vi "Ch_data_pattern_8_save (SubVI).vi"(7 "error in":errorcluster, 14 "T Cluster":T2 {"T8" format="%#.3f"; "T7" format="%#.3f"; "T6" format="%#.3f"; "T5" format="%#.3f"; "T4" format="%#.3f"; "T3" format="%#.3f"; "T2" format="%#.3f"; "T1" format="%#.3f"}, 17 "file":refnum<file>, 18 "R cluster":T1 {"R8" format="%#.3f"; "R7" format="%#.3f"; "R6" format="%#.3f"; "R5" format="%#.3f"; "R4" format="%#.3f"; "R3" format="%#.3f"; "R2" format="%#.3f"; "R1" format="%#.3f"}) -> (27 "error out":errorcluster)   [LabVIEW 2015]
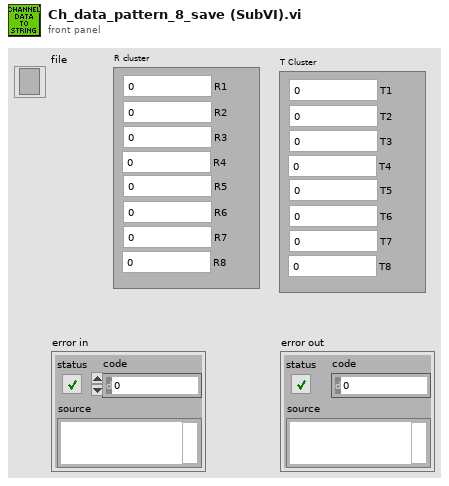
[diagram p1: front panel]
types:
  T1 = cluster{"R1":dbl, "R2":dbl, "R3":dbl, "R4":dbl, "R5":dbl, "R6":dbl, "R7":dbl, "R8":dbl}
  T2 = cluster{"T1":dbl, "T2":dbl, "T3":dbl, "T4":dbl, "T5":dbl, "T6":dbl, "T7":dbl, "T8":dbl}
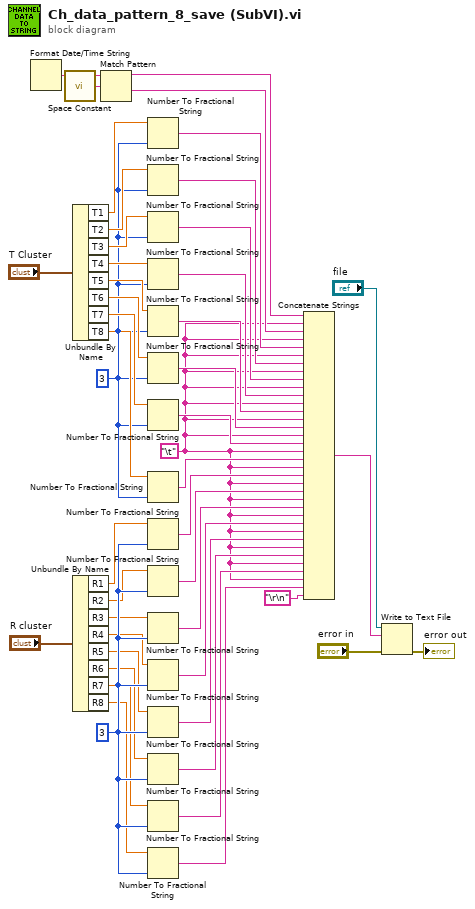
[diagram p0: block diagram]
diagram:
  w19 = i16 3 ("precision (6)")
  w25 = i16 3 ("precision (6)")
  w3 = "\t"
  n1 = Format Date/Time String() -> (date/time string=w44:string)  [unwired: 3 out]
  n2 = call <vilib>:"Space Constant.vi"() -> ("String"=w45:string)
  n3 = Unbundle By Name("T Cluster") -> ("T1"=w33:dbl, "T2"=w32:dbl, "T3"=w31:dbl, "T4"=w30:dbl, "T5"=w29:dbl, "T6"=w28:dbl, "T7"=w27:dbl, "T8"=w26:dbl)
  n4 = Unbundle By Name("R cluster") -> ("R1"=w18:dbl, "R2"=w17:dbl, "R3"=w16:dbl, "R4"=w15:dbl, "R5"=w14:dbl, "R6"=w13:dbl, "R7"=w12:dbl, "R8"=w11:dbl)
  n5 = Match Pattern(string=w44, regular expression=w45) -> (before substring=w37:string, after substring=w36:string)  [unwired: 3 out]
  n6 = Number To Fractional String(number=w33, precision (6)=w25) -> (F-format string=w42:string)  [unwired: 2 out]
  n7 = Number To Fractional String(number=w32, precision (6)=w25) -> (F-format string=w38:string)  [unwired: 2 out]
  n8 = Number To Fractional String(number=w31, precision (6)=w25) -> (F-format string=w41:string)  [unwired: 2 out]
  n9 = Number To Fractional String(number=w30, precision (6)=w25) -> (F-format string=w40:string)  [unwired: 2 out]
  n10 = Number To Fractional String(number=w29, precision (6)=w25) -> (F-format string=w24:string)  [unwired: 2 out]
  n11 = Number To Fractional String(number=w28, precision (6)=w25) -> (F-format string=w23:string)  [unwired: 2 out]
  n12 = Number To Fractional String(number=w27, precision (6)=w25) -> (F-format string=w22:string)  [unwired: 2 out]
  n13 = Number To Fractional String(number=w26, precision (6)=w25) -> (F-format string=w21:string)  [unwired: 2 out]
  n14 = Number To Fractional String(number=w18, precision (6)=w19) -> (F-format string=w10:string)  [unwired: 2 out]
  n15 = Number To Fractional String(number=w17, precision (6)=w19) -> (F-format string=w9:string)  [unwired: 2 out]
  n16 = Number To Fractional String(number=w16, precision (6)=w19) -> (F-format string=w8:string)  [unwired: 2 out]
  n17 = Number To Fractional String(number=w15, precision (6)=w19) -> (F-format string=w7:string)  [unwired: 2 out]
  n18 = Number To Fractional String(number=w14, precision (6)=w19) -> (F-format string=w6:string)  [unwired: 2 out]
  n19 = Number To Fractional String(number=w13, precision (6)=w19) -> (F-format string=w5:string)  [unwired: 2 out]
  n20 = Number To Fractional String(number=w12, precision (6)=w19) -> (F-format string=w4:string)  [unwired: 2 out]
  n21 = Number To Fractional String(number=w11, precision (6)=w19) -> (F-format string=w2:string)  [unwired: 2 out]
  n22 = Concatenate Strings(w37, w3, w36, w3, w42, w3, w38, w3, w41, w3, w40, w3, w24, w3, w23, w3, w22, w3, w21, w3, w10, w3, w9, w3, w8, w3, w7, w3, w6, w3, w5, w3, w4, w3, w2, "\r\n") -> (w35:string)
  n23 = Write to Text File(file (use dialog)="file", text=w35, error in="error in") -> (error out=→"error out":errorcluster)  [unwired: 3 out]
